vi "Pay.vi"(8 "error in (no error)":errorcluster, 10 "Accoounts":T1(c390), 11 "AIncome in":refnum<class "AIncome.lvclass">) -> (0 "error out":errorcluster, 2 "Accoounts out":T1(c390), 3 "AIncome out":refnum<class "AIncome.lvclass">)   [LabVIEW 2020, in "AIncome.lvclass"]
uses:
  AIncome.lvclass
  AIncome.lvclass/AIncome.ctl
  IBasicAccount/IBasicAccount.lvclass
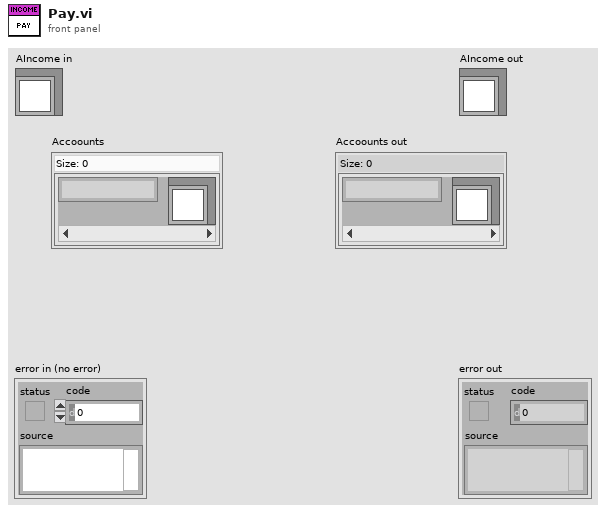
[diagram p1: front panel]
types:
  T1 = map{string, refnum<class "IBasicAccount.lvclass">}
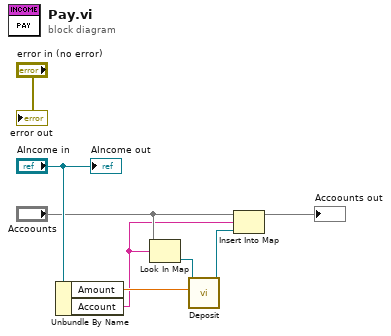
[diagram p0: block diagram]
diagram:
  n1 = Unbundle By Name("AIncome in") -> ("Amount"=w5:dbl, "Account"=w3:string)
  n2 = Look In Map(map="Accoounts", key=w3) -> (value=w6:refnum<class "IBasicAccount.lvclass">)  [unwired: 1 in, 1 out]
  n3 = call-dynamic "Deposit.vi"("Amount"=w5, "IDepositable in"=w6) -> ("IDepositable out"=w2:refnum<class "IBasicAccount.lvclass">)  [unwired: 7 in, 2 out]
  n4 = Insert Into Map(map in="Accoounts", key=w3, value=w2) -> (map out=→"Accoounts out":T1)  [unwired: 2 out]
  "error out" <- "error in (no error)"
  "AIncome out" <- "AIncome in"
